vi "Get Measurement Status.vi"(8 "error in (no error)":errorcluster, 10 "Measurement.lvclass":refnum<class "Measurement.lvclass">, 11 "Results in":refnum<class "Results.lvclass">) -> (0 "error out":errorcluster, 3 "Results out":refnum<class "Results.lvclass">)   [LabVIEW 2017, in "Result Actor.lvlib" / "Results.lvclass"]
uses:
  Results.lvclass
  Measurement Actor/Measurement.lvclass
  Controller/Unique Measurement ID.ctl
  Measurement Actor/Measurement.lvclass/Measurement.ctl
  Results.lvclass/Results.ctl
  Controller/Controller.lvclass
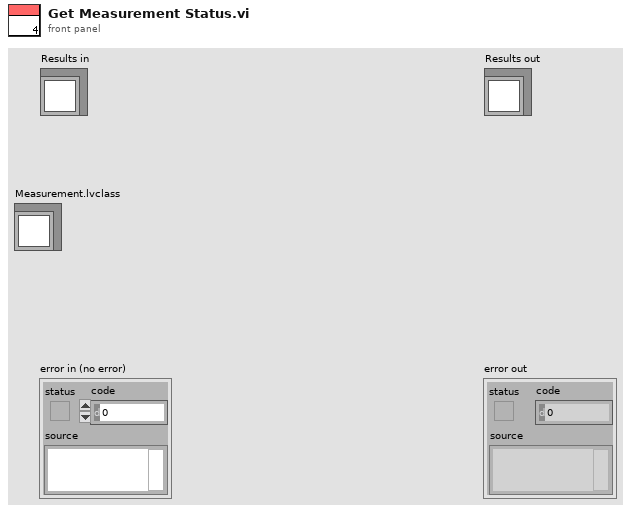
[diagram p1: front panel]
types:
  T1 = typedef "Controller Actor.lvlib/Controller.lvclass/Unique Measurement ID.ctl" = cluster{"Measurement Name":string, "Device Names":string[]}
  T2 = cluster{"Measurement Name":string, "Device Names":string[], "Time Stamp":timestamp}
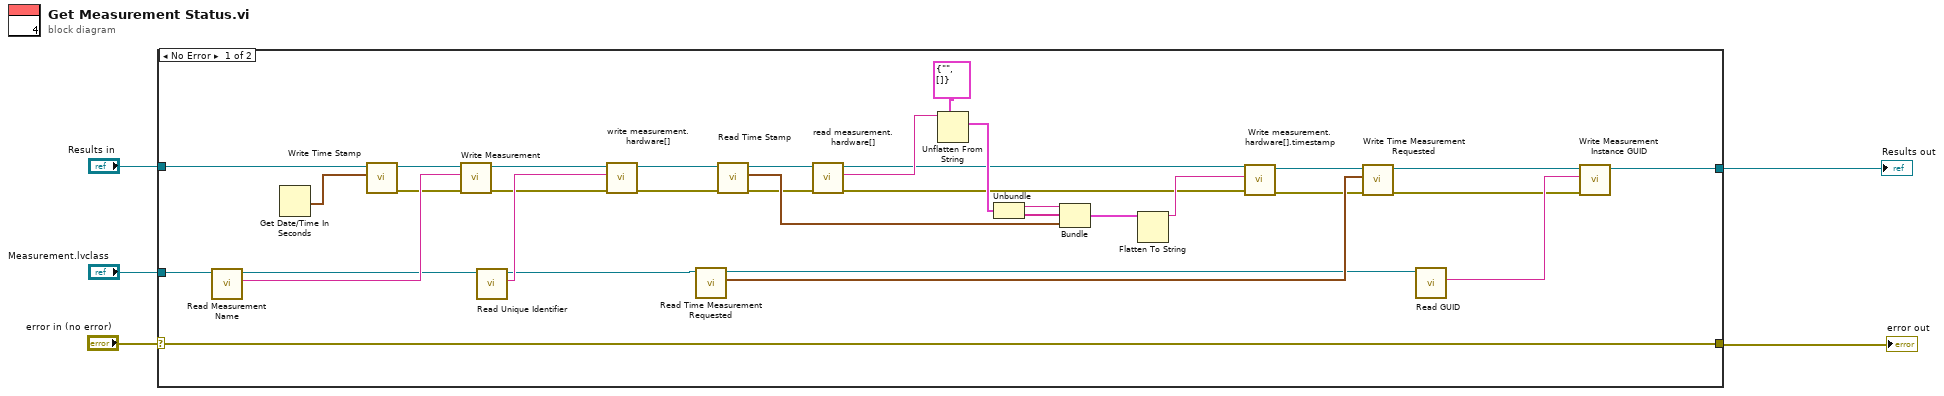
[diagram p0: block diagram]
diagram:
  n1 = case shown="No Error" "error in (no error)" {
    selector: "error in (no error)" -> [w39 w41]
    tunnel: [w39 w41] -> w4
    tunnel: [w14 w40] -> w2
    tunnel: "Results in" -> [w36 w40]
    tunnel: "Measurement.lvclass" -> [w34 _]
    frame No Error {
      n2 = call "Read Measurement Name.vi"("Measurement in"=w34) -> ("Measurement Name"=w35:string, "Measurement out"=w32:refnum<class "Measurement.lvclass">)  [unwired: 8 in, 1 out]
      n3 = Get Date/Time In Seconds() -> (seconds since 1Jan1904=w38:timestamp)
      n4 = call "Write Time Stamp.vi"("Time Stamp"=w38, "Results in"=w36) -> ("error out"=w12:errorcluster, "Results out"=w37:refnum<class "Results.lvclass">)  [unwired: 8 in]
      n5 = call "Write Measurement.vi"("error in (no error)"=w12, "Measurement"=w35, "Results in"=w37) -> ("error out"=w11:errorcluster, "Results out"=w33:refnum<class "Results.lvclass">)  [unwired: 7 in]
      n6 = call "Read Unique Identifier.vi"("Measurement in"=w32) -> ("Unique Identifier"=w31:string, "Measurement out"=w17:refnum<class "Measurement.lvclass">)  [unwired: 8 in, 1 out]
      n7 = call "write measurement.hardware[].vi"("error in (no error)"=w11, "uniqueid"=w31, "Results in"=w33) -> ("error out"=w10:errorcluster, "Results out"=w22:refnum<class "Results.lvclass">)  [unwired: 7 in]
      n8 = call "Read Time Measurement Requested.vi"("Measurement in"=w17) -> ("Time Measurement Requested"=w16:timestamp, "Measurement out"=w15:refnum<class "Measurement.lvclass">)  [unwired: 8 in, 1 out]
      n9 = call "Read Time Stamp.vi"("error in (no error)"=w10, "Results in"=w22) -> ("error out"=w9:errorcluster, "Time Stamp"=w30:timestamp, "Results out"=w28:refnum<class "Results.lvclass">)  [unwired: 7 in]
      n10 = call "read measurement.hardware[].vi"("error in (no error)"=w9, "Results in"=w28) -> ("error out"=w8:errorcluster, "uniqueid"=w23:string, "Results out"=w20:refnum<class "Results.lvclass">)  [unwired: 7 in]
      n11 = Unflatten From String(type=T1 {"Measurement Name"="", "Device Names"=[]} ("output cluster"), binary string=w23) -> (value=w26:T1)  [unwired: 3 in, 2 out]
      n12 = Unbundle(w26) -> ("Measurement Name"=w25:string, "Device Names"=w24:string[])
      n13 = Bundle("Measurement Name"=w25, "Device Names"=w24, "Time Stamp"=w30) -> (w29:T2)  [unwired: 1 in]
      n14 = Flatten To String(anything=w29) -> (data string=w21:string)  [unwired: 3 in, 2 out]
      n15 = call "Write measurement.hardware[].timestamp.vi"("error in (no error)"=w8, "measurement.hardware[].timestamp"=w21, "Results in"=w20) -> ("error out"=w7:errorcluster, "Results out"=w19:refnum<class "Results.lvclass">)  [unwired: 7 in]
      n16 = call "Write Time Measurement Requested.vi"("error in (no error)"=w7, "Time Measurement Requested"=w16, "Results in"=w19) -> ("error out"=w6:errorcluster, "Results out"=w18:refnum<class "Results.lvclass">)  [unwired: 7 in]
      n17 = call "Read GUID.vi"("Measurement in"=w15) -> ("GUID"=w13:string)  [unwired: 8 in, 2 out]
      n18 = call "Write Measurement Instance GUID.vi"("error in (no error)"=w6, "Measurement Instance GUID"=w13, "Results in"=w18) -> ("Results out"=w14:refnum<class "Results.lvclass">)  [unwired: 7 in, 1 out]
    }
    frame Error {
    }
  }
  "error out" <- w4
  "Results out" <- w2
